vi "build data string.vi"(0 "Data in":dbl[](array[numeric]), 1 "String in":string[](array[string]), 3 "error constant 2":errorcluster) -> (7 "Data out":string, 10 "error constant":errorcluster)   [LabVIEW 2014, in "get_data_mapper.lvlib"]
uses:
  get_data_mapper.lvlib
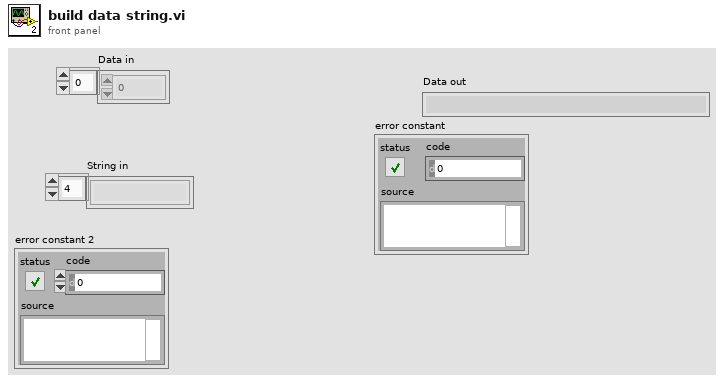
[diagram p1: front panel]
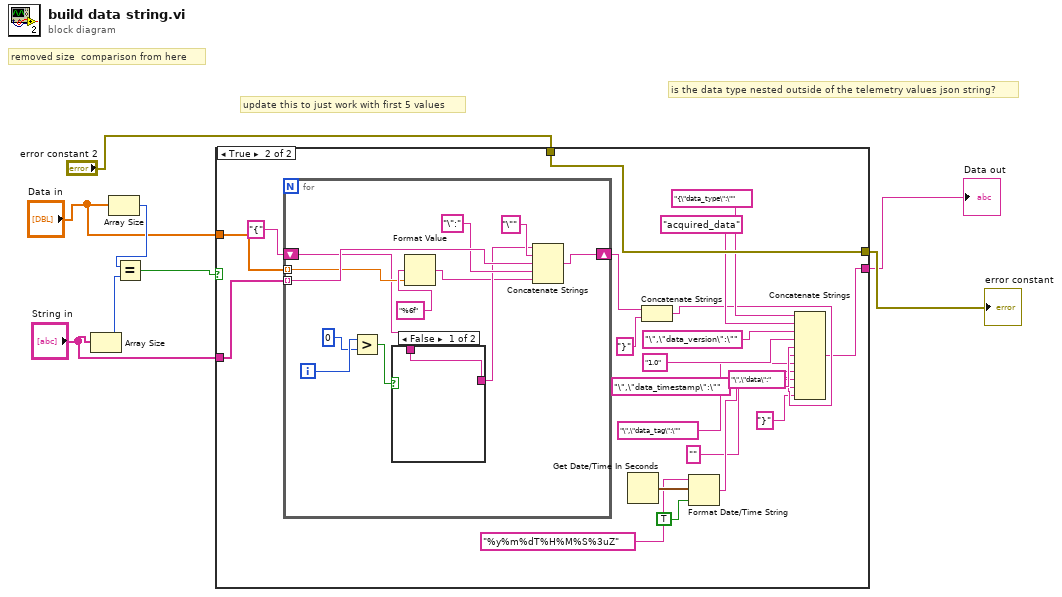
[diagram p0: block diagram]
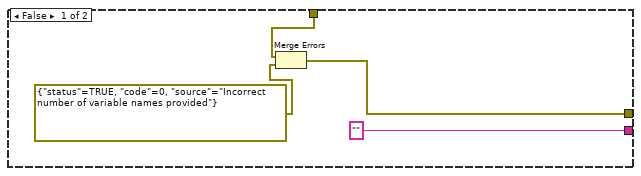
[diagram p2: hidden frame]
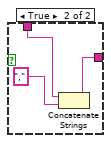
[diagram p3: hidden frame]
diagram:
  # "is the data type nested outside of the telemetry values json string?"
  # "removed size  comparison from here"
  # "update this to just work with first 5 values"
  n1 = Array Size(array="String in") -> (size(s)=w7:i32)
  n2 = Array Size(array="Data in") -> (size(s)=w8:i32)
  n3 = Equal?(x=w8, y=w7) -> (x = y?=w1:bool)
  n4 = case shown="True" w1 {
    tunnel: [w10 w28] -> w6
    tunnel: "String in" -> [_ w32]
    tunnel: ["" w13] -> w4
    tunnel: "Data in" -> [_ w31]
    tunnel: "error constant 2" -> [w11 w28]
    frame False {
      n5 = Merge Errors(w11, errorcluster {"status"=TRUE, "code"=0, "source"="Incorrect number of variable names provided"} ("error constant")) -> (w10:errorcluster)
    }
    frame True {
      n6 = for {
        shift-right: [w37] -> w30
        shift-left: "{" -> [w36]
        tunnel: w32 -> [w44] mode=indexing
        tunnel: w31 -> [w41] mode=indexing
        i -> [w40]
        n7 = Greater?(x=w40, y=0) -> (0:w38:bool)
        n8 = case shown="False" w38 {
          tunnel: w36 -> [w46 w49]
          tunnel: [w46 w47] -> w35
          frame False {
          }
          frame True {
            n9 = Concatenate Strings(w49, "," ("string")) -> (w47:string)
          }
        }
        n10 = Format Value(format string="%6f", value (0)=w41) -> (output string=w34:string)  [unwired: 1 in]
        n11 = Concatenate Strings(w35, "\"", w44, "\":", w34) -> (w37:string)
      }
      n12 = Get Date/Time In Seconds() -> (seconds since 1Jan1904=w22:timestamp)
      n13 = Concatenate Strings(w30, "}" ("string")) -> (w15:string)
      n14 = Format Date/Time String(time format string (%c)="%y%m%dT%H%M%S%3uZ", seconds (now)=w22, UTC format=TRUE) -> (date/time string=w19:string)
      n15 = Concatenate Strings("{\"data_type\":\"" ("string"), "acquired_data" ("string"), "\",\"data_version\":\"" ("string"), "1.0" ("string"), "\",\"data_timestamp\":\"" ("string"), w19, "\",\"data_tag\":\"" ("string"), "" ("string"), "\",\"data\":" ("string"), w15, "}" ("string")) -> (w13:string)
    }
  }
  "Data out" <- w4
  "error constant" <- w6
